vi "startReadManual.vi"(8 "error in (no error)":errorcluster, 10 "ElectrometerController in":refnum<class "ElectrometerController.lvclass">, 11 "State in":refnum<class "ElectrometerState.lvclass">) -> (0 "error out":errorcluster, 2 "ElectrometerController. out":refnum<class "ElectrometerController.lvclass">, 3 "State out":refnum<class "ElectrometerState.lvclass">)   [LabVIEW 2016, in "ElectrometerState.lvclass"]
uses:
  ElectrometerState.lvclass
  ElectrometerController/ElectrometerController.lvclass
  ts_electrometeruserevents/Typedefs/RejectedCommand.ctl
  ts_electrometeruserevents/Typedefs/CommandValue.ctl
  ts_electrometeruserevents/Typedefs/StateValue.ctl
  ts_electrometeruserevents/Typedefs/ElectrometerTypedefs.lvlib
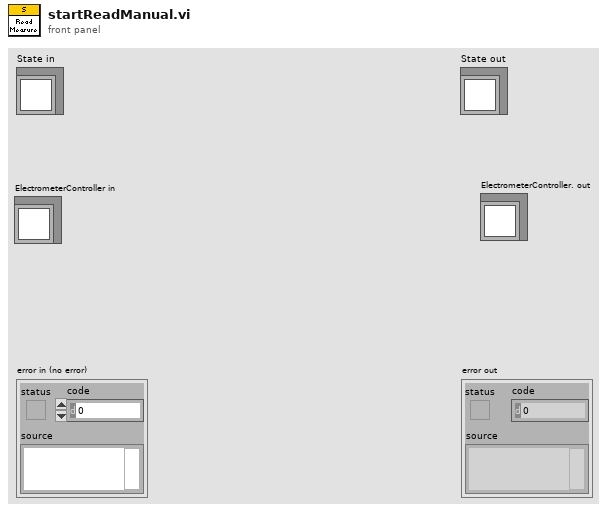
[diagram p1: front panel]
types:
  T1 = typedef "ElectrometerTypedefs.lvlib/RejectedCommand.ctl" = cluster{"CommandValue":T2, "StateValue":T3, "Time Stamp":dbl}
  T2 = typedef "ElectrometerTypedefs.lvlib/CommandValue.ctl" = enum16{"ClearError", "Disable", "Enable", "Exit", "GoToStandby", "OnHeartbeat", "OnIncomingMessagingError", "OnInterrupt", "Start", "SetDigitalFilter", "StartScan", "StartScanDt", "StartScanReachIntensity", "StopScan", "SetIntegrationTime", "PerformZeroCalib", "SetRange", "SetMode", "Power"}
  T3 = typedef "ElectrometerTypedefs.lvlib/StateValue.ctl" = enum16{"OffState", "StandbyState", "DisabledState", "EnabledState", "FaultState", "SetDurationReadingState", "ConfiguringState", "ReadyState", "ManualReadingState", "UntilIntentisyReadingState"}
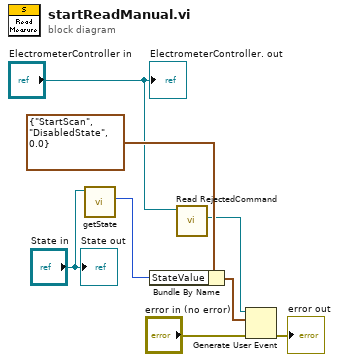
[diagram p0: block diagram]
diagram:
  n1 = call-dynamic "getState.vi"("State in"="State in") -> ("StateValue"=w6:T3)  [unwired: 8 in, 2 out]
  n2 = Bundle By Name(cluster=T1 {"CommandValue"=enum."StartScan", "StateValue"=enum."DisabledState", "Time Stamp"=0.0} ("event data"), "StateValue"=w6) -> (w7:T1)
  n3 = call-dynamic "Read RejectedCommand.vi"("ElectrometerController in"="ElectrometerController in") -> ("RejectedCommand"=w1:refnum<user-event>)  [unwired: 8 in, 2 out]
  n4 = Generate User Event(user event=w1, event data cluster=w7, error in="error in (no error)") -> (error out=→"error out":errorcluster)  [unwired: 1 in, 1 out]
  "State out" <- "State in"
  "ElectrometerController. out" <- "ElectrometerController in"
